vi "SetErrorControl.vi"(8 "error in (no error)":errorcluster, 9 "error":errorcluster, 10 "Name":string, 11 "VIEW in":refnum<class "VIEW.lvclass">) -> (0 "error out":errorcluster, 3 "VIEW out":refnum<class "VIEW.lvclass">)   [LabVIEW 2013, in "VIEW.lvclass"]
uses:
  VIEW.lvclass
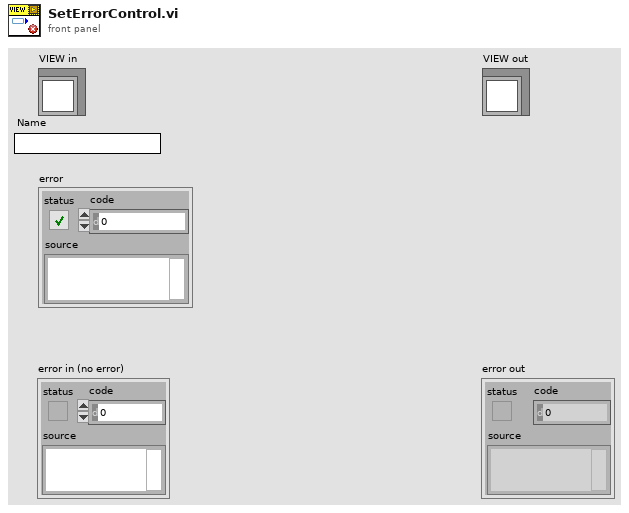
[diagram p1: front panel]
types:
  T1 = cluster{"CtlRef":refnum<vi>, "Name":string, "ClassName":string}
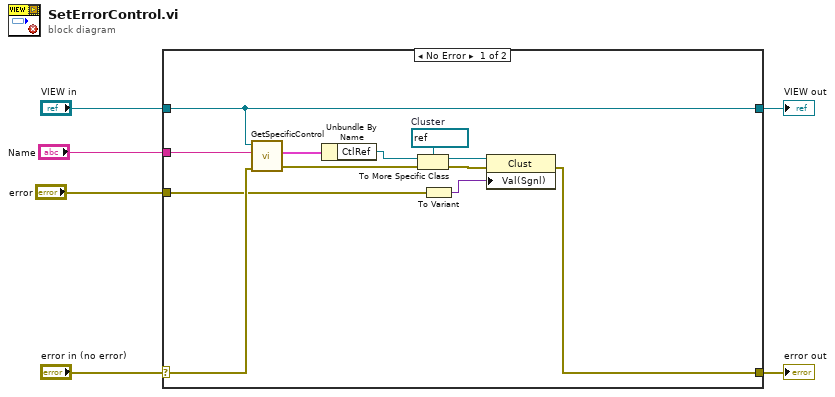
[diagram p0: block diagram]
diagram:
  n1 = case shown="No Error" "error in (no error)" {
    selector: "error in (no error)" -> [w13 w20]
    tunnel: [w9 w20] -> w5
    tunnel: [w18 w19] -> w3
    tunnel: "VIEW in" -> [w18 w19]
    tunnel: "Name" -> [w17 _]
    tunnel: "error" -> [w8 _]
    frame No Error {
      w12 = refnum<vi> refnum  # Cluster
      n2 = call "GetSpecificControl.vi"("error in (no error)"=w13, "Name"=w17, "VIEW in"=w18) -> ("error out"=w14:errorcluster, "output cluster"=w15:T1)  [unwired: 6 in, 1 out]
      n3 = Unbundle By Name(w15) -> ("CtlRef"=w16:refnum<vi>)
      n4 = To More Specific Class(target class=w12, reference=w16, error in=w14) -> (specific class reference=w11:refnum<vi>, error out=w10:errorcluster)
      n5 = To Variant(anything=w8) -> (Variant=w7:variant)
      n6 = property class="Clust"(reference=w11, error in=w10, "Val(Sgnl)"=w7) -> (error out=w9:errorcluster)  [unwired: 1 out]
    }
    frame Error {
    }
  }
  "error out" <- w5
  "VIEW out" <- w3
